vi "step_moves.vi"(9 "Changelist":T4[](array[typedef]), 10 "Board Layout":cluster{"Piece Type":T1, "Team Color":T2}[][](array[cluster]), 11 "Team Color":T2) -> (2 "New Board Layout":cluster{"Piece Type":T1, "Team Color":T2}[][](array[cluster]), 3 "Movelist":T3[](array[typedef]))   [LabVIEW 2015]
uses:
  chess_poschangeinfo_cluster.ctl
  chess_piecetype_enum.ctl
  chess_teamcolor_enum.ctl
  chess_moveinfo_cluster.ctl
panel:
  in  "move info def":T3
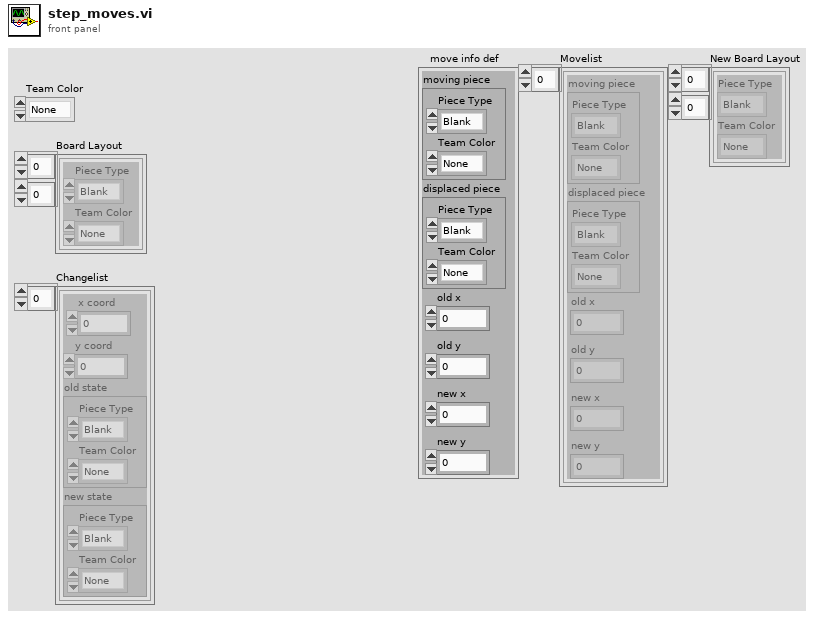
[diagram p1: front panel]
types:
  T1 = typedef "chess_piecetype_enum.ctl" = enum16{"Blank", "Pawn", "Rook", "Knight", "Bishop", "Queen", "King"}
  T2 = typedef "chess_teamcolor_enum.ctl" = enum16{"None", "Red", "Blue"}
  T3 = typedef "chess_moveinfo_cluster.ctl" = cluster{"moving piece":cluster{"Piece Type":T1, "Team Color":T2}, "displaced piece":cluster{"Piece Type":T1, "Team Color":T2}, "old x":i32, "old y":i32, "new x":i32, "new y":i32}
  T4 = typedef "chess_poschangeinfo_cluster.ctl" = cluster{"x coord":i32, "y coord":i32, "old state":cluster{"Piece Type":T1, "Team Color":T2}, "new state":cluster{"Piece Type":T1, "Team Color":T2}}
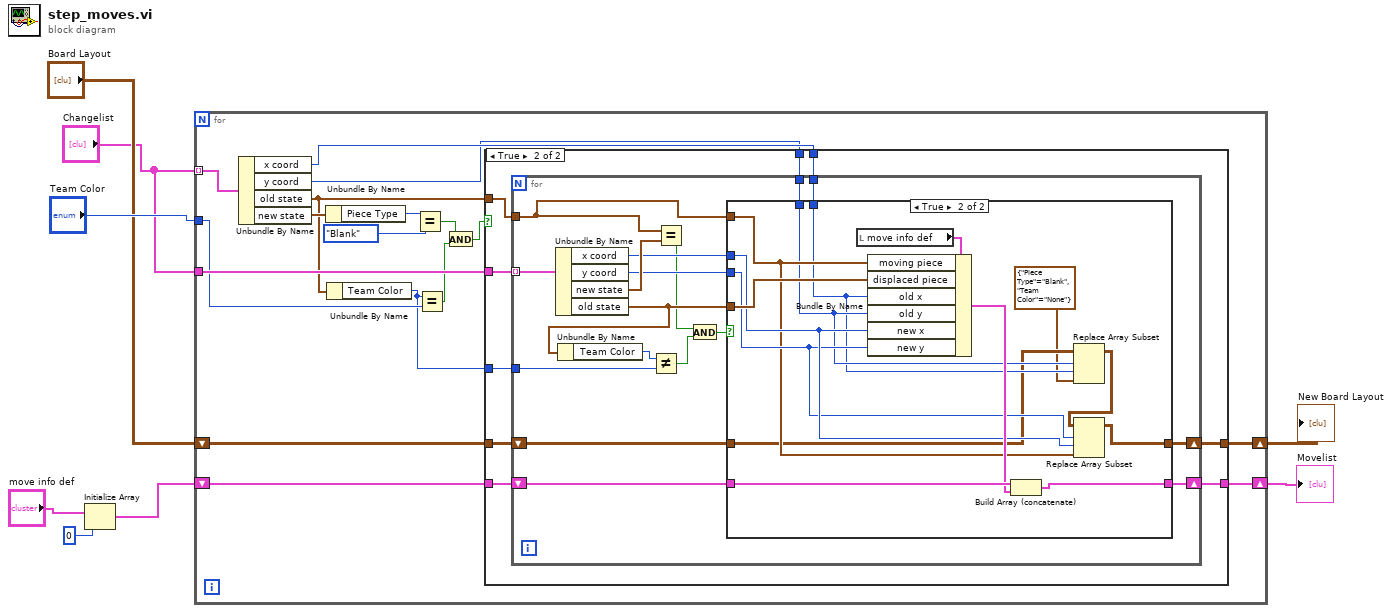
[diagram p0: block diagram]
diagram:
  n1 = Initialize Array("move info def", 0 ("dimension size")) -> (w4:T3[])
  n2 = for {
    tunnel: "Team Color" -> [w19]
    tunnel: "Changelist" -> [w25] mode=indexing
    shift-right: [w13] -> w2
    shift-left: w4 -> [w12]
    tunnel: "Changelist" -> [w21]
    shift-right: [w10] -> w1
    shift-left: "Board Layout" -> [w11]
    n3 = Unbundle By Name(w25) -> ("x coord"=w15:i32, "y coord"=w14:i32, "old state"=w20:cluster{"Piece Type":T1, "Team Color":T2}, "new state"=w24:cluster{"Piece Type":T1, "Team Color":T2})
    n4 = Unbundle By Name(w24) -> ("Piece Type"=w23:T1)
    n5 = Unbundle By Name(w20) -> ("Team Color"=w9:T2)
    n6 = Equal?(x=w23, y=chess_piecetype_enum."Blank") -> (x = y?=w18:bool)
    n7 = Equal?(x=w9, y=w19) -> (x = y?=w17:bool)
    n8 = And(x=w18, y=w17) -> (x .and. y?=w16:bool)
    n9 = case shown="True" w16 {
      tunnel: w21 -> [_ w36]
      tunnel: w20 -> [_ w35]
      tunnel: w15 -> [_ w34]
      tunnel: w14 -> [_ w33]
      tunnel: [w27 w32] -> w13
      tunnel: w12 -> [w27 w31]
      tunnel: w11 -> [w26 w30]
      tunnel: [w26 w29] -> w10
      tunnel: w9 -> [_ w28]
      frame False {
      }
      frame True {
        n10 = for {
          tunnel: w36 -> [w53] mode=indexing
          tunnel: w35 -> [w37]
          tunnel: w34 -> [w51]
          tunnel: w33 -> [w50]
          shift-right: [w47] -> w32
          shift-left: w31 -> [w46]
          shift-right: [w44] -> w29
          shift-left: w30 -> [w45]
          tunnel: w28 -> [w41]
          n11 = Unbundle By Name(w53) -> ("x coord"=w49:i32, "y coord"=w48:i32, "new state"=w52:cluster{"Piece Type":T1, "Team Color":T2}, "old state"=w43:cluster{"Piece Type":T1, "Team Color":T2})
          n12 = Unbundle By Name(w43) -> ("Team Color"=w42:T2)
          n13 = Not Equal?(x=w42, y=w41) -> (x != y?=w39:bool)
          n14 = Equal?(x=w37, y=w52) -> (x = y?=w40:bool)
          n15 = And(x=w40, y=w39) -> (x .and. y?=w38:bool)
          n16 = case shown="True" w38 {
            tunnel: w43 -> [_ w68]
            tunnel: w37 -> [_ w61]
            tunnel: w51 -> [_ w59]
            tunnel: w50 -> [_ w60]
            tunnel: w49 -> [_ w63]
            tunnel: w48 -> [_ w62]
            tunnel: [w55 w67] -> w47
            tunnel: w46 -> [w55 w66]
            tunnel: w45 -> [w54 w58]
            tunnel: [w54 w64] -> w44
            frame False {
            }
            frame True {
              n17 = local read "move info def"() -> (w69:T3)
              n18 = Bundle By Name(cluster=w69, "moving piece"=w61, "displaced piece"=w68, "old x"=w59, "old y"=w60, "new x"=w63, "new y"=w62) -> (w65:T3)
              n19 = Build Array (concatenate)(w66, w65) -> (w67:T3[])
              n20 = Replace Array Subset(array=w58, new element=cluster{"Piece Type":T1, "Team Color":T2} {"Piece Type"=enum."Blank", "Team Color"=enum."None"} ("new element/subarray"), index (row)=w60, index (col)=w59) -> (w57:cluster{"Piece Type":T1, "Team Color":T2}[][])
              n21 = Replace Array Subset(array=w57, new element=w61, index (row)=w62, index (col)=w63) -> (w64:cluster{"Piece Type":T1, "Team Color":T2}[][])
            }
          }
        }
      }
    }
  }
  "Movelist" <- w2
  "New Board Layout" <- w1
